vi "Shift.vi"() -> ()   [LabVIEW 2017]
uses:
  <vilib>/addons/database/Connection.llb/DB Tools Open Connec (String).vi
  <vilib>/addons/database/Auxilliary.llb/DB Tools Format Datetime String (Time Stamp).vi
  Global/Global 1.vi
  <vilib>/addons/database/NI_Database_API.lvlib
panel:
  out "error out":errorcluster
  in  "Cycle_time(s)":dbl
  out "x-y":dbl
  out "x-y 8":dbl
  out "x-y 7":dbl
  in  "INCLUDED 9":bool=TRUE
  in  "INCLUDED 8":bool=TRUE
  in  "INCLUDED 7":bool=TRUE
  in  "INCLUDED 6":bool=TRUE
  in  "INCLUDED 5":bool=TRUE
  in  "INCLUDED 4":bool=TRUE
  in  "INCLUDED 3":bool=TRUE
  in  "INCLUDED 2":bool=TRUE
  in  "INCLUDED":bool=TRUE
  in  "EXTRA SHIFT INCLUDED":bool=TRUE
  in  "Cancel Button":bool
  in  "Save Button":bool
  in  "Cluster 12":T1 {"1Start 4" format="%<%H:%M:%S>T"; "1Start 3" format="%<%H:%M:%S>T"; "1Start 2" format="%<%H:%M:%S>T"; "1Start" format="%<%H:%M:%S>T"}
  in  "Cluster 11":T1 {"1Start 4" format="%<%H:%M:%S>T"; "1Start 3" format="%<%H:%M:%S>T"; "1Start 2" format="%<%H:%M:%S>T"; "1Start" format="%<%H:%M:%S>T"}
  in  "Cluster 10":T1 {"1Start 4" format="%<%H:%M:%S>T"; "1Start 3" format="%<%H:%M:%S>T"; "1Start 2" format="%<%H:%M:%S>T"; "1Start" format="%<%H:%M:%S>T"}
  in  "Cluster 9":T1 {"1Start 4" format="%<%H:%M:%S>T"; "1Start 3" format="%<%H:%M:%S>T"; "1Start 2" format="%<%H:%M:%S>T"; "1Start" format="%<%H:%M:%S>T"}
  in  "Cluster 8":T2 {"1Start 8" format="%<%H:%M:%S>T"; "1Start 7" format="%<%H:%M:%S>T"; "1Start 6" format="%<%H:%M:%S>T"; "1Start 5" format="%<%H:%M:%S>T"; "1Start 4" format="%<%H:%M:%S>T"; "1Start 3" format="%<%H:%M:%S>T"; "1Start 2" format="%<%H:%M:%S>T"; "1Start" format="%<%H:%M:%S>T"}
  in  "Cluster 7":T2 {"1Start 8" format="%<%H:%M:%S>T"; "1Start 7" format="%<%H:%M:%S>T"; "1Start 6" format="%<%H:%M:%S>T"; "1Start 5" format="%<%H:%M:%S>T"; "1Start 4" format="%<%H:%M:%S>T"; "1Start 3" format="%<%H:%M:%S>T"; "1Start 2" format="%<%H:%M:%S>T"; "1Start" format="%<%H:%M:%S>T"}
  in  "Cluster 6":T2 {"1Start 8" format="%<%H:%M:%S>T"; "1Start 7" format="%<%H:%M:%S>T"; "1Start 6" format="%<%H:%M:%S>T"; "1Start 5" format="%<%H:%M:%S>T"; "1Start 4" format="%<%H:%M:%S>T"; "1Start 3" format="%<%H:%M:%S>T"; "1Start 2" format="%<%H:%M:%S>T"; "1Start" format="%<%H:%M:%S>T"}
  in  "Cluster 5":T2 {"1Start 8" format="%<%H:%M:%S>T"; "1Start 7" format="%<%H:%M:%S>T"; "1Start 6" format="%<%H:%M:%S>T"; "1Start 5" format="%<%H:%M:%S>T"; "1Start 4" format="%<%H:%M:%S>T"; "1Start 3" format="%<%H:%M:%S>T"; "1Start 2" format="%<%H:%M:%S>T"; "1Start" format="%<%H:%M:%S>T"}
  in  "Blank Button":bool
  in  "Cluster 4":T3 {"1Start 6" format="%<%H:%M:%S>T"; "1Start 5" format="%<%H:%M:%S>T"; "1Start 4" format="%<%H:%M:%S>T"; "1Start 3" format="%<%H:%M:%S>T"; "1Start 2" format="%<%H:%M:%S>T"; "1Start" format="%<%H:%M:%S>T"}
  in  "Cluster 3":T3 {"1Start 6" format="%<%H:%M:%S>T"; "1Start 5" format="%<%H:%M:%S>T"; "1Start 4" format="%<%H:%M:%S>T"; "1Start 3" format="%<%H:%M:%S>T"; "1Start 2" format="%<%H:%M:%S>T"; "1Start" format="%<%H:%M:%S>T"}
  in  "Cluster 2":T3 {"1Start 2" format="%<%H:%M:%S>T"; "1Start" format="%<%H:%M:%S>T"; "1Start 6" format="%<%H:%M:%S>T"; "1Start 5" format="%<%H:%M:%S>T"; "1Start 4" format="%<%H:%M:%S>T"; "1Start 3" format="%<%H:%M:%S>T"}
  in  "Cluster":T3 {"1Start 6" format="%<%H:%M:%S>T"; "1Start 5" format="%<%H:%M:%S>T"; "1Start 4" format="%<%H:%M:%S>T"; "1Start 3" format="%<%H:%M:%S>T"; "1Start 2" format="%<%H:%M:%S>T"; "1Start" format="%<%H:%M:%S>T"}
  # "SHIFT SETTING"
  # "EXTRA SHIFT"
  # "X"
  # "Y"
  # "A"
  # "B"
  # "C"
  # "D"
  # "BREAK 3"
  # "START"
  # "END"
  # "BREAK 2"
  # "START"
  # "END"
  # "BREAK 1"
  # "START"
  # "END"
  # "SHIFT IN DAY"
  # "CODE"
  # "START"
  # "END"
  # "A"
  # "B"
  # "C"
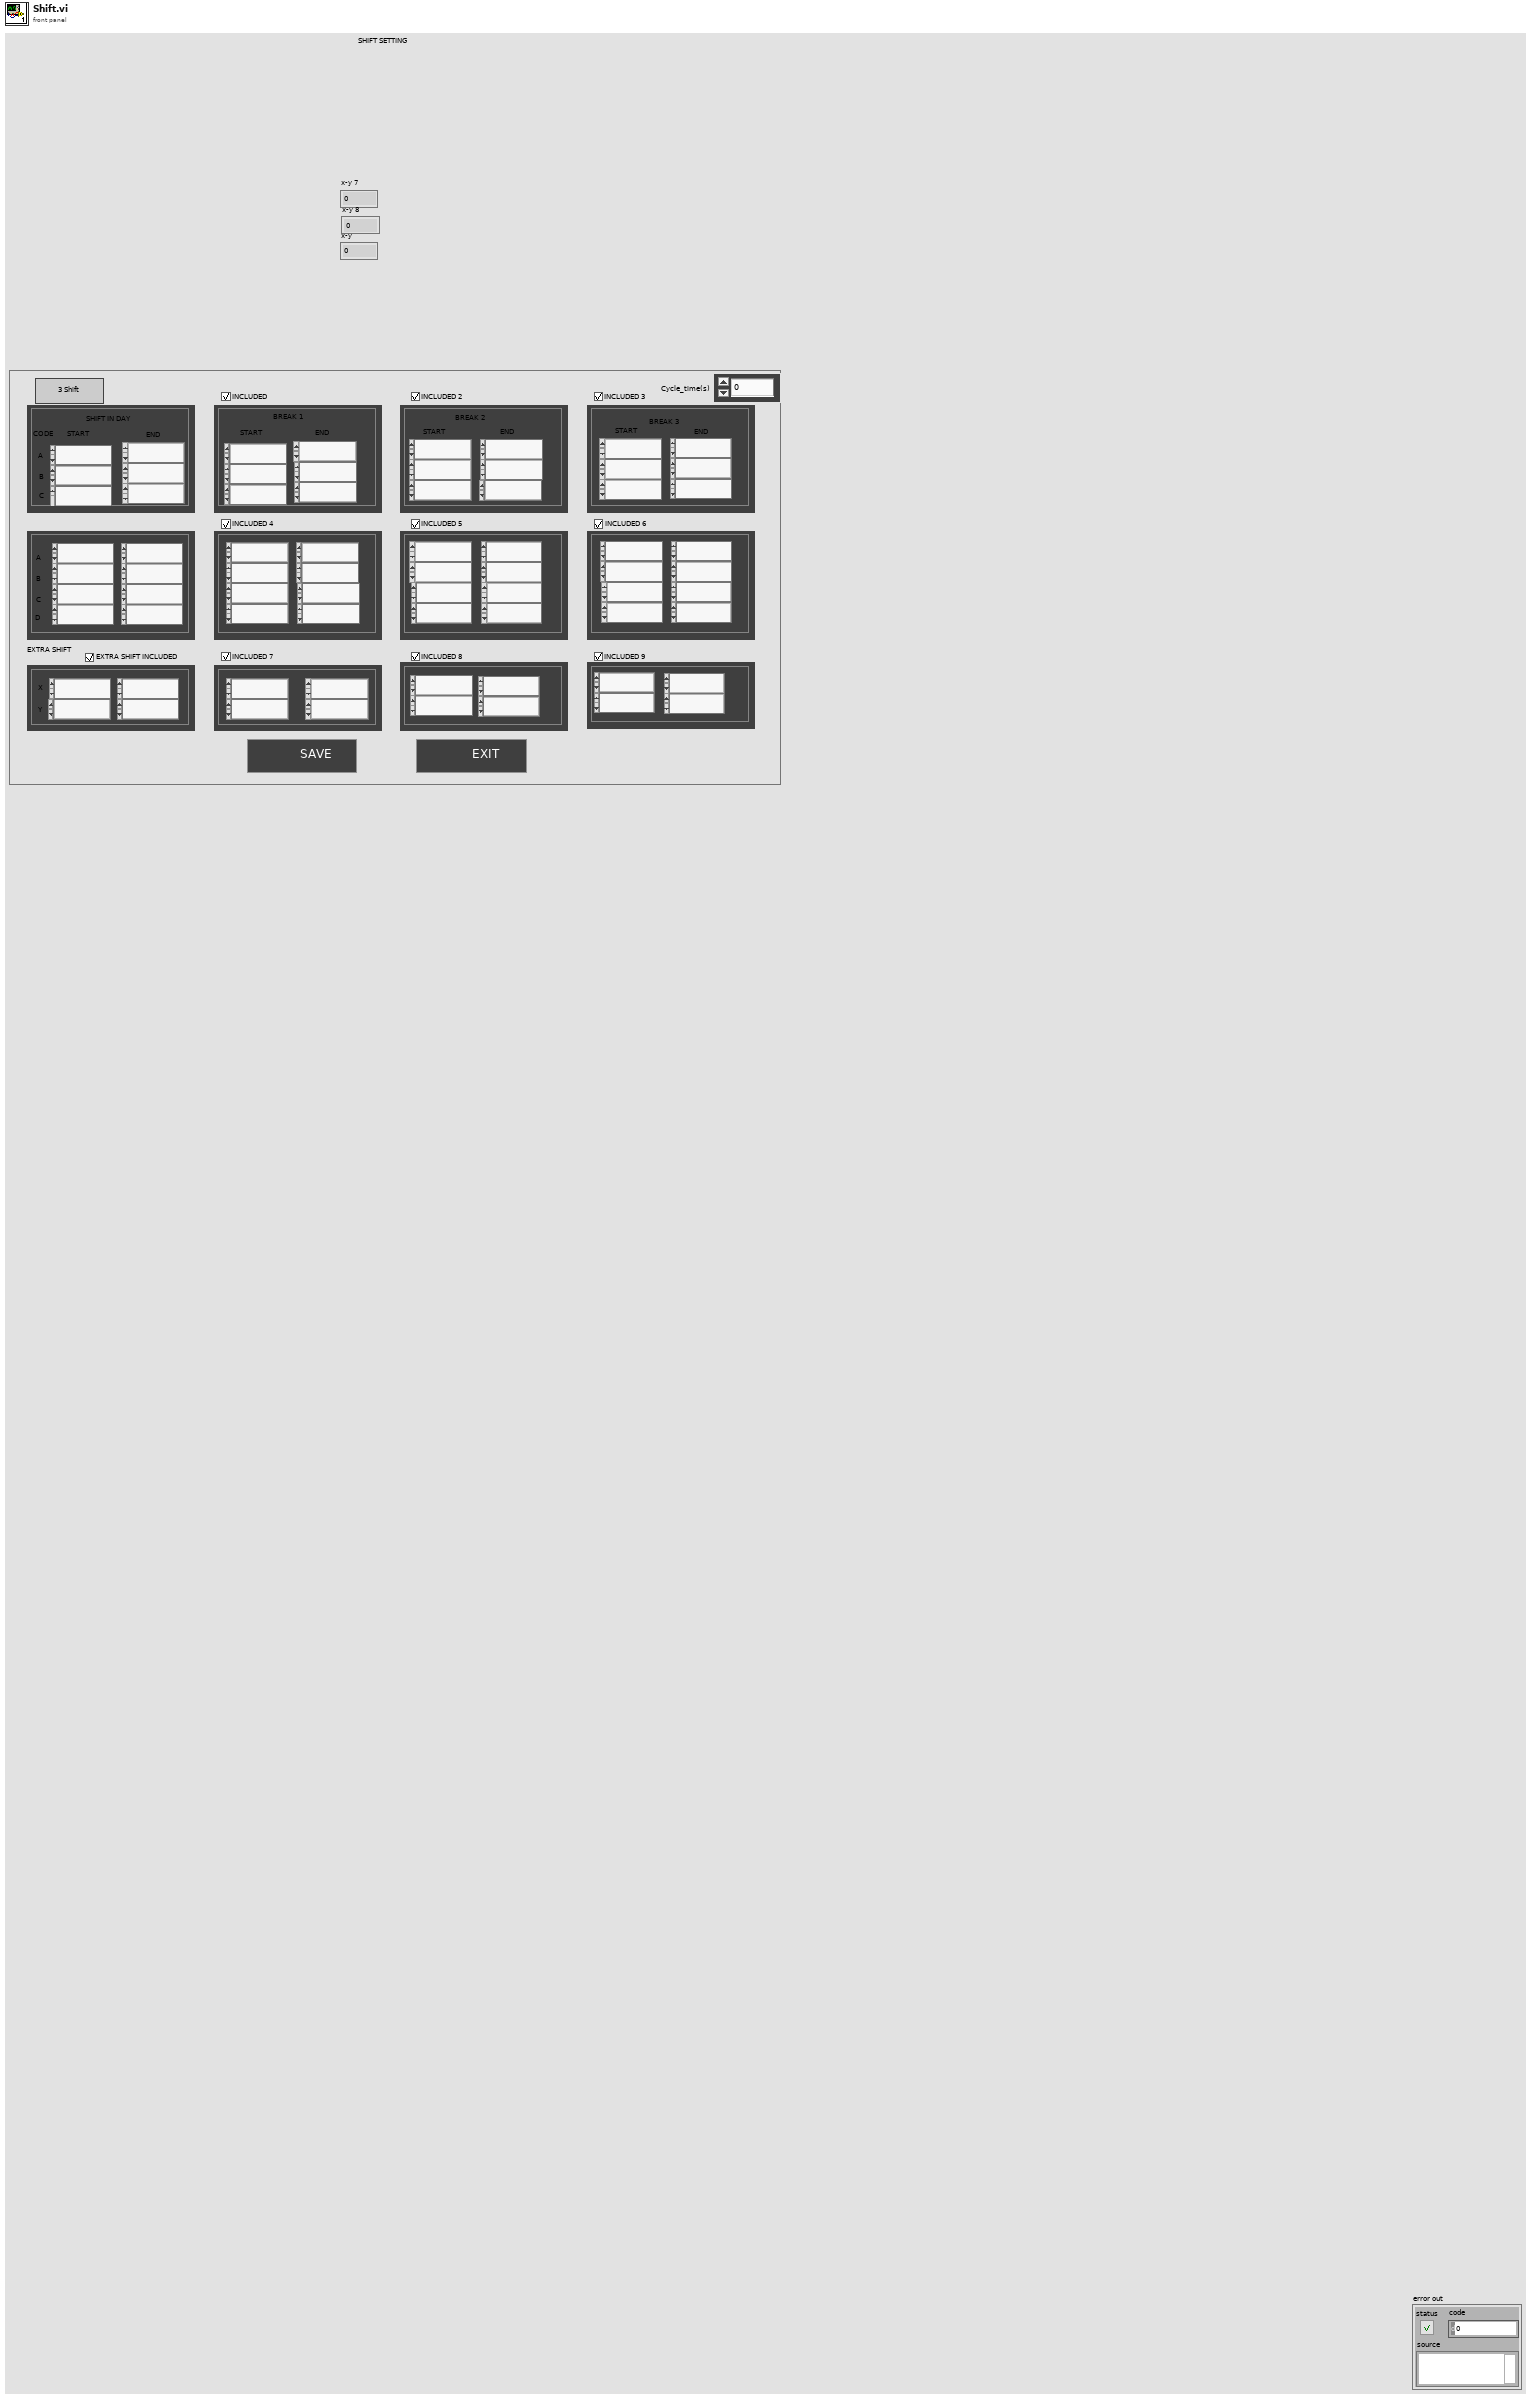
[diagram p1: front panel]
types:
  T1 = cluster{"1Start":timestamp, "1Start 2":timestamp, "1Start 3":timestamp, "1Start 4":timestamp}
  T2 = cluster{"1Start":timestamp, "1Start 2":timestamp, "1Start 3":timestamp, "1Start 4":timestamp, "1Start 5":timestamp, "1Start 6":timestamp, "1Start 7":timestamp, "1Start 8":timestamp}
  T3 = cluster{"1Start":timestamp, "1Start 2":timestamp, "1Start 3":timestamp, "1Start 4":timestamp, "1Start 5":timestamp, "1Start 6":timestamp}
  T4 = typedef "NI_Database_API.lvlib/Conn ObjectReference.ctl" = refnum<k1>
  T5 = cluster{"Time Stamp Out[0]":timestamp, "Time Stamp Out[1]":timestamp, "Time Stamp Out[2]":timestamp, "Time Stamp Out[3]":timestamp, "Time Stamp Out[4]":timestamp, "Time Stamp Out[5]":timestamp}
  T6 = cluster{"Time Stamp Out[0]":timestamp, "Time Stamp Out[1]":timestamp, "Time Stamp Out[2]":timestamp, "Time Stamp Out[3]":timestamp}
  T7 = cluster{"Time Stamp Out[0]":timestamp, "Time Stamp Out[1]":timestamp, "Time Stamp Out[2]":timestamp, "Time Stamp Out[3]":timestamp, "Time Stamp Out[4]":timestamp, "Time Stamp Out[5]":timestamp, "Time Stamp Out[6]":timestamp, "Time Stamp Out[7]":timestamp}
  T8 = cluster{"INCLUDED 9":bool, "date/time string":string, "date/time string":string, "date/time string":string, "date/time string":string}
  T9 = cluster{"INCLUDED 7":bool, "date/time string":string, "date/time string":string, "date/time string":string, "date/time string":string}
  T10 = cluster{"EXTRA SHIFT INCLUDED":bool, "date/time string":string, "date/time string":string, "date/time string":string, "date/time string":string}
  T11 = cluster{"INCLUDED 8":bool, "date/time string":string, "date/time string":string, "date/time string":string, "date/time string":string}
  T12 = cluster{"Blank Button":bool, "date/time string":string, "date/time string":string, "date/time string":string, "date/time string":string, "date/time string":string, "date/time string":string}
  T13 = cluster{"INCLUDED":bool, "date/time string":string, "date/time string":string, "date/time string":string, "date/time string":string, "date/time string":string, "date/time string":string}
  T14 = cluster{"INCLUDED 4":bool, "date/time string":string, "date/time string":string, "date/time string":string, "date/time string":string, "date/time string":string, "date/time string":string, "date/time string":string, "date/time string":string}
  T15 = cluster{"date/time string":string, "date/time string":string, "date/time string":string, "date/time string":string, "date/time string":string, "date/time string":string, "date/time string":string, "date/time string":string}
  T16 = cluster{"INCLUDED 6":bool, "date/time string":string, "date/time string":string, "date/time string":string, "date/time string":string, "date/time string":string, "date/time string":string, "date/time string":string, "date/time string":string}
  T17 = cluster{"INCLUDED 5":bool, "date/time string":string, "date/time string":string, "date/time string":string, "date/time string":string, "date/time string":string, "date/time string":string, "date/time string":string, "date/time string":string}
  T18 = cluster{"INCLUDED 2":bool, "date/time string":string, "date/time string":string, "date/time string":string, "date/time string":string, "date/time string":string, "date/time string":string}
  T19 = cluster{"INCLUDED 3":bool, "date/time string":string, "date/time string":string, "date/time string":string, "date/time string":string, "date/time string":string, "date/time string":string}
  T20 = enum32{"invalid app kind", "Development System", "Run Time System", "Student Edition", "Embedded LabVIEW", "Evaluation", "Custom"}
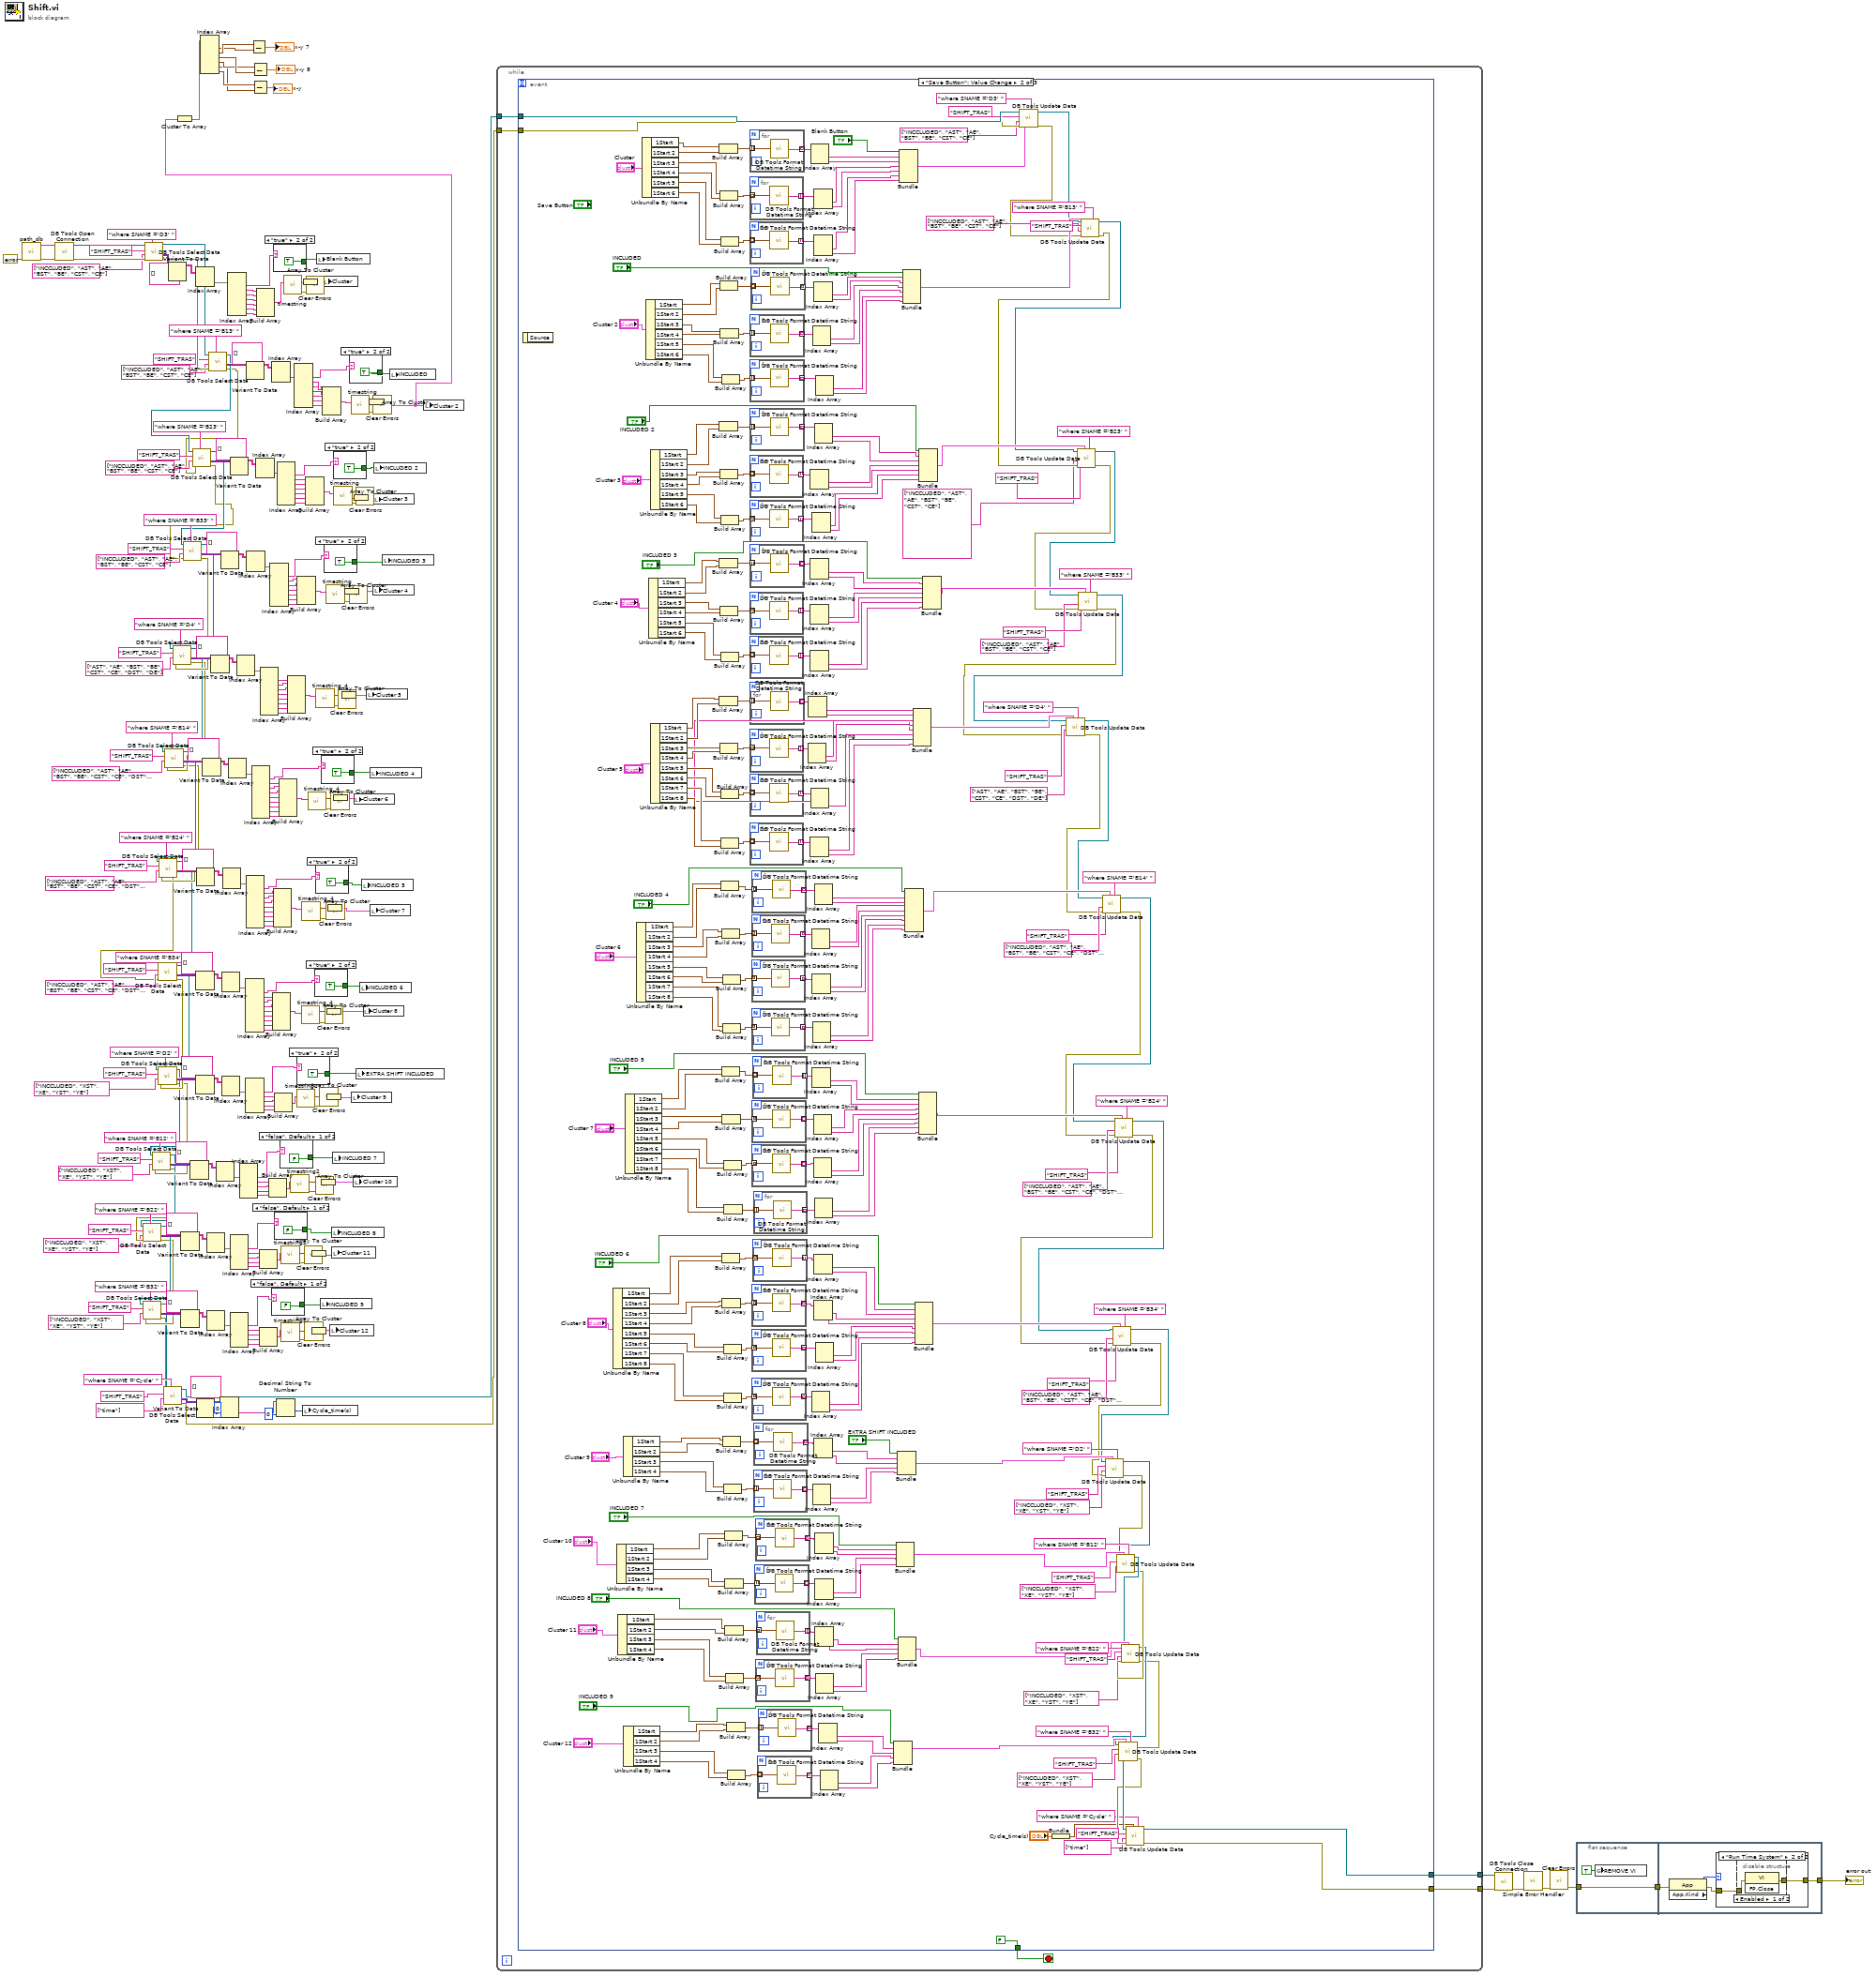
[diagram p0: block diagram]
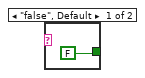
[diagram p4: hidden frame]
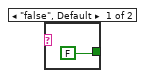
[diagram p5: hidden frame]
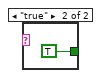
[diagram p6: hidden frame]
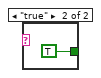
[diagram p7: hidden frame]
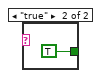
[diagram p8: hidden frame]
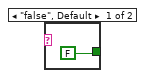
[diagram p9: hidden frame]
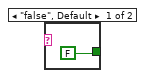
[diagram p10: hidden frame]
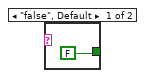
[diagram p11: hidden frame]
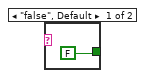
[diagram p12: hidden frame]
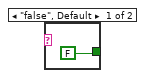
[diagram p13: hidden frame]
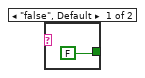
[diagram p14: hidden frame]
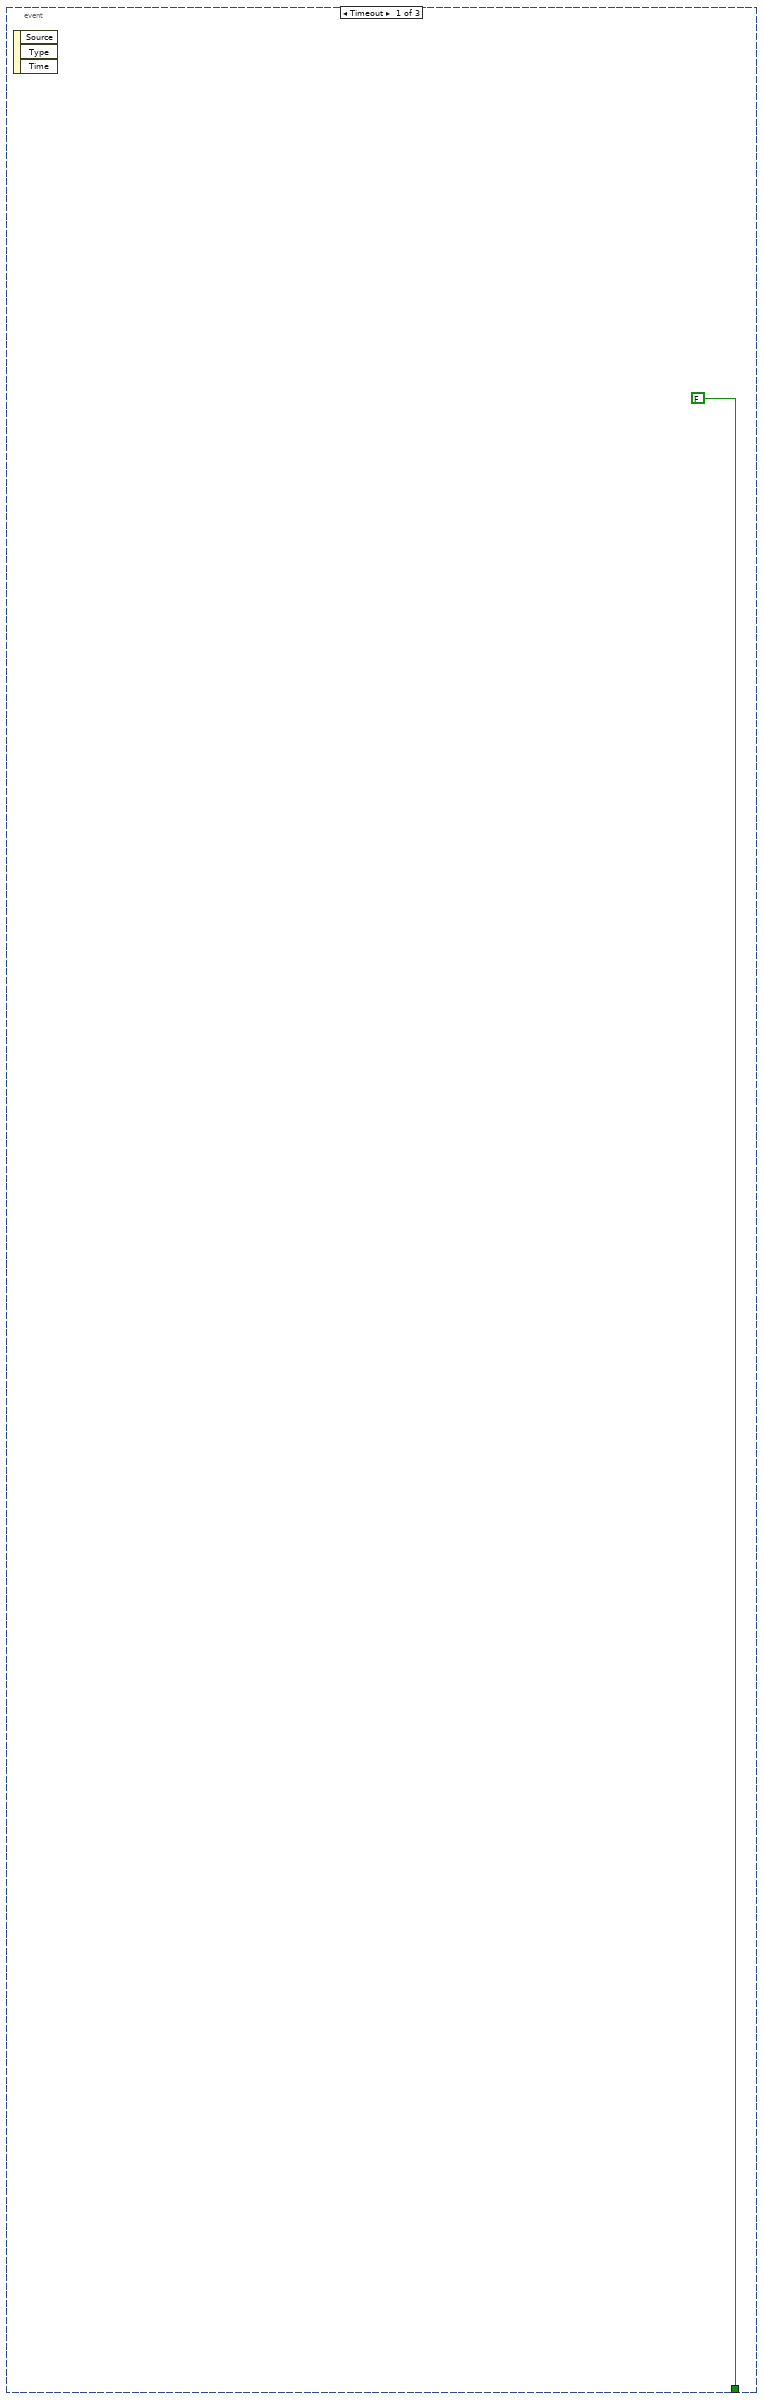
[diagram p15: hidden frame]
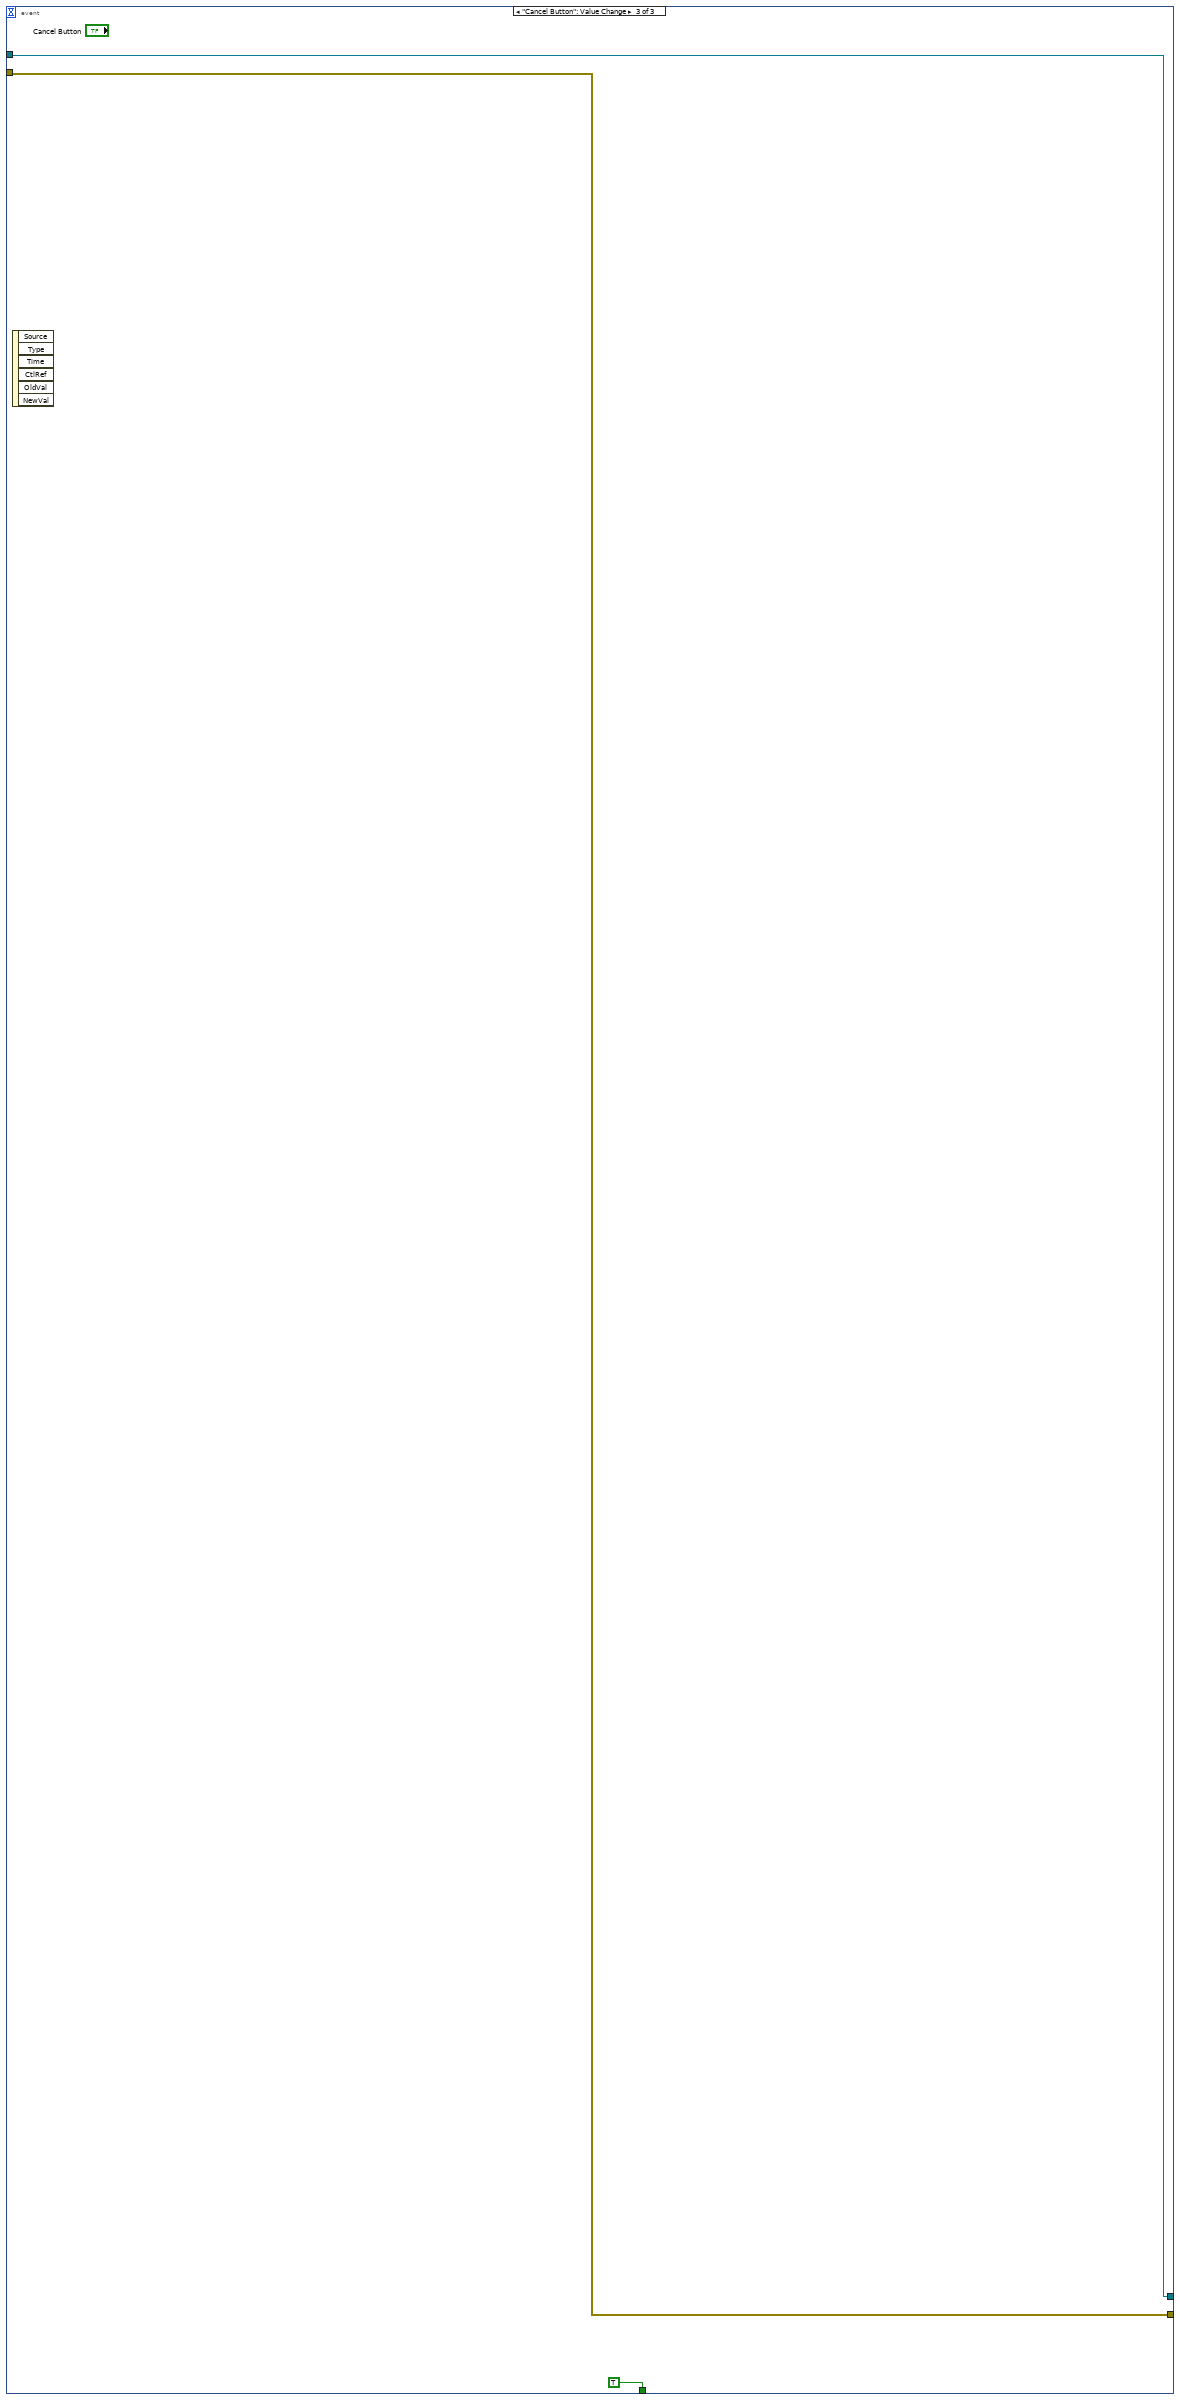
[diagram p16: hidden frame]
diagram:
  n1 = call "path_db.vi"("error in"=errorcluster {"status"=FALSE, "code"=0, "source"=""}) -> ("error out"=w284:errorcluster, "resulting string"=w285:string)  [unwired: 9 in]
  n2 = call-poly <vilib>:"DB Tools Open Connection.vi"("error in (no error)"=w284, "connection information"=w285) -> ("error out"=w281:errorcluster, "connection reference"=w280:T4)  [unwired: 6 in]
  n3 = call <vilib>:"DB Tools Select Data.vi"("condition"="where SNAME ='D3' ", "error in (no error)"=w281, "columns"=string[] ["INCCLUDED", "AST", "AE", "BST", "BE", "CST", "CE"], "table"="SHIFT_TRAS", "connection reference"=w280) -> ("error out"=w272:errorcluster, "data"=w277:variant[][], "connection reference out"=w271:T4)  [unwired: 1 in]
  n4 = Variant To Data(type=string[][] [], Variant=w277) -> (data=w275:string[][])  [unwired: 1 in, 1 out]
  n5 = Index Array(array=w275) -> (element=w43:string[])  [unwired: 2 in]
  n6 = call <vilib>:"DB Tools Select Data.vi"("condition"="where SNAME ='B13' ", "error in (no error)"=w272, "columns"=string[] ["INCCLUDED", "AST", "AE", "BST", "BE", "CST", "CE"], "table"="SHIFT_TRAS", "connection reference"=w271) -> ("error out"=w62:errorcluster, "data"=w267:variant[][], "connection reference out"=w217:T4)  [unwired: 1 in]
  n7 = call <vilib>:"DB Tools Select Data.vi"("condition"="where SNAME ='B23' ", "error in (no error)"=w62, "columns"=string[] ["INCCLUDED", "AST", "AE", "BST", "BE", "CST", "CE"], "table"="SHIFT_TRAS", "connection reference"=w217) -> ("error out"=w215:errorcluster, "data"=w241:variant[][], "connection reference out"=w216:T4)  [unwired: 1 in]
  n8 = call <vilib>:"DB Tools Select Data.vi"("condition"="where SNAME ='B33' ", "error in (no error)"=w215, "columns"=string[] ["INCCLUDED", "AST", "AE", "BST", "BE", "CST", "CE"], "table"="SHIFT_TRAS", "connection reference"=w216) -> ("error out"=w195:errorcluster, "data"=w234:variant[][], "connection reference out"=w196:T4)  [unwired: 1 in]
  n9 = call <vilib>:"DB Tools Select Data.vi"("condition"="where SNAME ='D4' ", "error in (no error)"=w195, "columns"=string[] ["AST", "AE", "BST", "BE", "CST", "CE", "DST", "DE"], "table"="SHIFT_TRAS", "connection reference"=w196) -> ("error out"=w75:errorcluster, "data"=w203:variant[][], "connection reference out"=w76:T4)  [unwired: 1 in]
  n10 = call <vilib>:"DB Tools Select Data.vi"("condition"="where SNAME ='B14' ", "error in (no error)"=w75, "columns"=string[] ["INCCLUDED", "AST", "AE", "BST", "BE", "CST", "CE", "DST", "DE"], "table"="SHIFT_TRAS", "connection reference"=w76) -> ("error out"=w73:errorcluster, "data"=w190:variant[][], "connection reference out"=w74:T4)  [unwired: 1 in]
  n11 = call <vilib>:"DB Tools Select Data.vi"("condition"="where SNAME ='B24' ", "error in (no error)"=w73, "columns"=string[] ["INCCLUDED", "AST", "AE", "BST", "BE", "CST", "CE", "DST", "DE"], "table"="SHIFT_TRAS", "connection reference"=w74) -> ("error out"=w71:errorcluster, "data"=w161:variant[][], "connection reference out"=w72:T4)  [unwired: 1 in]
  n12 = call <vilib>:"DB Tools Select Data.vi"("condition"="where SNAME ='B34' ", "error in (no error)"=w71, "columns"=string[] ["INCCLUDED", "AST", "AE", "BST", "BE", "CST", "CE", "DST", "DE"], "table"="SHIFT_TRAS", "connection reference"=w72) -> ("error out"=w69:errorcluster, "data"=w152:variant[][], "connection reference out"=w70:T4)  [unwired: 1 in]
  n13 = call <vilib>:"DB Tools Select Data.vi"("condition"="where SNAME ='D2' ", "error in (no error)"=w69, "columns"=string[] ["INCCLUDED", "XST", "XE", "YST", "YE"], "table"="SHIFT_TRAS", "connection reference"=w70) -> ("error out"=w67:errorcluster, "data"=w129:variant[][], "connection reference out"=w68:T4)  [unwired: 1 in]
  n14 = call <vilib>:"DB Tools Select Data.vi"("condition"="where SNAME ='B12' ", "error in (no error)"=w67, "columns"=string[] ["INCCLUDED", "XST", "XE", "YST", "YE"], "table"="SHIFT_TRAS", "connection reference"=w68) -> ("error out"=w65:errorcluster, "data"=w115:variant[][], "connection reference out"=w66:T4)  [unwired: 1 in]
  n15 = call <vilib>:"DB Tools Select Data.vi"("condition"="where SNAME ='B22' ", "error in (no error)"=w65, "columns"=string[] ["INCCLUDED", "XST", "XE", "YST", "YE"], "table"="SHIFT_TRAS", "connection reference"=w66) -> ("error out"=w63:errorcluster, "data"=w104:variant[][], "connection reference out"=w64:T4)  [unwired: 1 in]
  n16 = call <vilib>:"DB Tools Select Data.vi"("condition"="where SNAME ='B32' ", "error in (no error)"=w63, "columns"=string[] ["INCCLUDED", "XST", "XE", "YST", "YE"], "table"="SHIFT_TRAS", "connection reference"=w64) -> ("error out"=w14:errorcluster, "data"=w91:variant[][], "connection reference out"=w15:T4)  [unwired: 1 in]
  n17 = call <vilib>:"DB Tools Select Data.vi"("condition"="where SNAME ='Cycle' ", "error in (no error)"=w14, "columns"=string[] ["time"], "table"="SHIFT_TRAS", "connection reference"=w15) -> ("error out"=w13:errorcluster, "data"=w19:variant[][], "connection reference out"=w12:T4)  [unwired: 1 in]
  n18 = Variant To Data(type=string[][] [], Variant=w104) -> (data=w106:string[][])  [unwired: 1 in, 1 out]
  n19 = Variant To Data(type=string[][] [], Variant=w91) -> (data=w89:string[][])  [unwired: 1 in, 1 out]
  n20 = Variant To Data(type=string[][] [], Variant=w115) -> (data=w113:string[][])  [unwired: 1 in, 1 out]
  n21 = Variant To Data(type=string[][] [], Variant=w152) -> (data=w150:string[][])  [unwired: 1 in, 1 out]
  n22 = Variant To Data(type=string[][] [], Variant=w129) -> (data=w131:string[][])  [unwired: 1 in, 1 out]
  n23 = Variant To Data(type=string[][] [], Variant=w161) -> (data=w163:string[][])  [unwired: 1 in, 1 out]
  n24 = Variant To Data(type=string[][] [], Variant=w19) -> (data=w17:string[][])  [unwired: 1 in, 1 out]
  n25 = Variant To Data(type=string[][] [], Variant=w190) -> (data=w188:string[][])  [unwired: 1 in, 1 out]
  n26 = Index Array(array=w106) -> (element=w107:string[])  [unwired: 2 in]
  n27 = Index Array(array=w89) -> (element=w88:string[])  [unwired: 2 in]
  n28 = Variant To Data(type=string[][] [], Variant=w203) -> (data=w205:string[][])  [unwired: 1 in, 1 out]
  n29 = Index Array(array=w113) -> (element=w112:string[])  [unwired: 2 in]
  n30 = Index Array(array=w17, index (row)=0, index (col)=0 ("disabled index (col)")) -> (element=w9:string)
  n31 = Variant To Data(type=string[][] [], Variant=w234) -> (data=w232:string[][])  [unwired: 1 in, 1 out]
  n32 = Index Array(array=w150) -> (element=w149:string[])  [unwired: 2 in]
  n33 = Index Array(array=w131) -> (element=w132:string[])  [unwired: 2 in]
  n34 = Index Array(array=w163) -> (element=w164:string[])  [unwired: 2 in]
  n35 = Index Array(array=w43) -> (element #1=w35:string, element #2=w41:string, element #3=w40:string, element #4=w39:string, element #5=w38:string, element #6=w37:string, element #7=w36:string)  [unwired: 7 in]
  n36 = Index Array(array=w188) -> (element=w187:string[])  [unwired: 2 in]
  n37 = Variant To Data(type=string[][] [], Variant=w241) -> (data=w243:string[][])  [unwired: 1 in, 1 out]
  n38 = Index Array(array=w107) -> (element #1=w84:string, element #2=w100:string, element #3=w101:string, element #4=w99:string, element #5=w98:string)  [unwired: 5 in]
  n39 = Index Array(array=w88) -> (element #1=w83:string, element #2=w95:string, element #3=w94:string, element #4=w96:string, element #5=w97:string)  [unwired: 5 in]
  n40 = Index Array(array=w205) -> (element=w206:string[])  [unwired: 2 in]
  n41 = Index Array(array=w112) -> (element #1=w85:string, element #2=w119:string, element #3=w118:string, element #4=w120:string, element #5=w121:string)  [unwired: 5 in]
  n42 = Index Array(array=w149) -> (element #1=w139:string, element #2=w156:string, element #3=w148:string, element #4=w147:string, element #5=w146:string, element #6=w145:string, element #7=w144:string, element #8=w143:string, element #9=w155:string)  [unwired: 9 in]
  n43 = Index Array(array=w132) -> (element #1=w45:string, element #2=w125:string, element #3=w126:string, element #4=w123:string, element #5=w122:string)  [unwired: 5 in]
  n44 = Variant To Data(type=string[][] [], Variant=w267) -> (data=w265:string[][])  [unwired: 1 in, 1 out]
  n45 = Index Array(array=w164) -> (element #1=w174:string, element #2=w157:string, element #3=w165:string, element #4=w166:string, element #5=w167:string, element #6=w168:string, element #7=w169:string, element #8=w170:string, element #9=w158:string)  [unwired: 9 in]
  n46 = Index Array(array=w232) -> (element=w231:string[])  [unwired: 2 in]
  n47 = Index Array(array=w187) -> (element #1=w176:string, element #2=w194:string, element #3=w186:string, element #4=w185:string, element #5=w184:string, element #6=w183:string, element #7=w182:string, element #8=w181:string, element #9=w193:string)  [unwired: 9 in]
  n48 = Index Array(array=w243) -> (element=w244:string[])  [unwired: 2 in]
  n49 = Build Array(w41, w40, w39, w38, w37, w36) -> (w42:string[])
  n50 = Build Array(w100, w101, w99, w98) -> (w108:string[])
  n51 = Build Array(w95, w94, w96, w97) -> (w87:string[])
  n52 = Index Array(array=w206) -> (element #1=w198:string, element #2=w207:string, element #3=w208:string, element #4=w209:string, element #5=w210:string, element #6=w211:string, element #7=w212:string, element #8=w199:string)  [unwired: 8 in]
  n53 = Build Array(w119, w118, w120, w121) -> (w111:string[])
  n54 = Index Array(array=w231) -> (element #1=w222:string, element #2=w230:string, element #3=w229:string, element #4=w228:string, element #5=w227:string, element #6=w226:string, element #7=w225:string)  [unwired: 7 in]
  n55 = Index Array(array=w265) -> (element=w264:string[])  [unwired: 2 in]
  n56 = case shown="\"false\", Default" w83 {
    tunnel: [FALSE TRUE] -> w78
    frame "false", Default {
    }
    frame "true" {
    }
  }
  n57 = Build Array(w156, w148, w147, w146, w145, w144, w143, w155) -> (w142:string[])
  n58 = case shown="\"true\"" w35 {
    tunnel: [FALSE TRUE] -> w34
    frame "false", Default {
    }
    frame "true" {
    }
  }
  n59 = Build Array(w157, w165, w166, w167, w168, w169, w170, w158) -> (w171:string[])
  n60 = Build Array(w125, w126, w123, w122) -> (w133:string[])
  n61 = case shown="\"false\", Default" w84 {
    tunnel: [FALSE TRUE] -> w80
    frame "false", Default {
    }
    frame "true" {
    }
  }
  n62 = Decimal String To Number(string=w9, offset=0) -> (number=w8:i32)  [unwired: 1 in, 1 out]
  n63 = Index Array(array=w244) -> (element #1=w253:string, element #2=w245:string, element #3=w246:string, element #4=w247:string, element #5=w248:string, element #6=w249:string, element #7=w250:string)  [unwired: 7 in]
  n64 = Build Array(w194, w186, w185, w184, w183, w182, w181, w193) -> (w180:string[])
  n65 = case shown="\"false\", Default" w85 {
    tunnel: [FALSE TRUE] -> w81
    frame "false", Default {
    }
    frame "true" {
    }
  }
  n66 = call "timestring2.vi"("String Array In"=w108) -> ("error out"=w57:errorcluster, "Time Stamp Out"=w109:timestamp[])  [unwired: 9 in]
  n67 = call "timestring2.vi"("String Array In"=w87) -> ("error out"=w58:errorcluster, "Time Stamp Out"=w86:timestamp[])  [unwired: 9 in]
  n68 = call "timestring.vi"("String Array In"=w42) -> ("error out"=w47:errorcluster, "Time Stamp Out"=w274:timestamp[])  [unwired: 9 in]
  n69 = Build Array(w198, w207, w208, w209, w210, w211, w212, w199) -> (w213:string[])
  n70 = call "timestring2.vi"("String Array In"=w111) -> ("error out"=w56:errorcluster, "Time Stamp Out"=w110:timestamp[])  [unwired: 9 in]
  n71 = Index Array(array=w264) -> (element #1=w255:string, element #2=w263:string, element #3=w262:string, element #4=w261:string, element #5=w260:string, element #6=w259:string, element #7=w258:string)  [unwired: 7 in]
  n72 = call "timestring2.vi"("String Array In"=w133) -> ("error out"=w55:errorcluster, "Time Stamp Out"=w134:timestamp[])  [unwired: 9 in]
  n73 = Build Array(w230, w229, w228, w227, w226, w225) -> (w224:string[])
  n74 = case shown="\"true\"" w45 {
    tunnel: [FALSE TRUE] -> w44
    frame "false", Default {
    }
    frame "true" {
    }
  }
  n75 = Array To Cluster(array=w274) -> (cluster=w273:T5)
  n76 = call "timestring_4.vi"("String Array In"=w142) -> ("error out"=w54:errorcluster, "Time Stamp Out"=w141:timestamp[])  [unwired: 9 in]
  n77 = call "timestring_4.vi"("String Array In"=w171) -> ("error out"=w53:errorcluster, "Time Stamp Out"=w172:timestamp[])  [unwired: 9 in]
  n78 = local write "Cycle_time(s)"(w8) -> ()
  n79 = call <vilib>:"Clear Errors.vi"("error in (no error)"=w57) -> ()  [unwired: 5 in, 2 out]
  n80 = call <vilib>:"Clear Errors.vi"("error in (no error)"=w58) -> ()  [unwired: 5 in, 2 out]
  n81 = Build Array(w245, w246, w247, w248, w249, w250) -> (w251:string[])
  n82 = call <vilib>:"Clear Errors.vi"("error in (no error)"=w47) -> ()  [unwired: 5 in, 2 out]
  n83 = call "timestring_4.vi"("String Array In"=w180) -> ("error out"=w52:errorcluster, "Time Stamp Out"=w179:timestamp[])  [unwired: 9 in]
  n84 = Array To Cluster(array=w109) -> (cluster=w79:T6)
  n85 = Array To Cluster(array=w86) -> (cluster=w77:T6)
  n86 = case shown="\"true\"" w139 {
    tunnel: [FALSE TRUE] -> w135
    frame "false", Default {
    }
    frame "true" {
    }
  }
  n87 = case shown="\"true\"" w174 {
    tunnel: [FALSE TRUE] -> w136
    frame "false", Default {
    }
    frame "true" {
    }
  }
  n88 = call <vilib>:"Clear Errors.vi"("error in (no error)"=w56) -> ()  [unwired: 5 in, 2 out]
  n89 = call "timestring_4.vi"("String Array In"=w213) -> ("error out"=w51:errorcluster, "Time Stamp Out"=w214:timestamp[])  [unwired: 9 in]
  n90 = local write "Blank Button"(w34) -> ()
  n91 = Array To Cluster(array=w110) -> (cluster=w82:T6)
  n92 = call <vilib>:"Clear Errors.vi"("error in (no error)"=w55) -> ()  [unwired: 5 in, 2 out]
  n93 = local write "INCLUDED 9"(w78) -> ()
  n94 = case shown="\"true\"" w176 {
    tunnel: [FALSE TRUE] -> w175
    frame "false", Default {
    }
    frame "true" {
    }
  }
  n95 = local write "Cluster"(w273) -> ()
  n96 = Build Array(w263, w262, w261, w260, w259, w258) -> (w257:string[])
  n97 = case shown="\"true\"" w222 {
    tunnel: [FALSE TRUE] -> w219
    frame "false", Default {
    }
    frame "true" {
    }
  }
  n98 = Array To Cluster(array=w141) -> (cluster=w137:T7)
  n99 = call <vilib>:"Clear Errors.vi"("error in (no error)"=w54) -> ()  [unwired: 5 in, 2 out]
  n100 = Array To Cluster(array=w134) -> (cluster=w124:T6)
  n101 = Array To Cluster(array=w172) -> (cluster=w138:T7)
  n102 = call "timestring.vi"("String Array In"=w224) -> ("error out"=w50:errorcluster, "Time Stamp Out"=w223:timestamp[])  [unwired: 9 in]
  n103 = call <vilib>:"Clear Errors.vi"("error in (no error)"=w53) -> ()  [unwired: 5 in, 2 out]
  n104 = local write "Cluster 12"(w77) -> ()
  n105 = call <vilib>:"Clear Errors.vi"("error in (no error)"=w52) -> ()  [unwired: 5 in, 2 out]
  n106 = Array To Cluster(array=w179) -> (cluster=w178:T7)
  n107 = local write "INCLUDED 8"(w80) -> ()
  n108 = local write "Cluster 11"(w79) -> ()
  n109 = local write "INCLUDED 7"(w81) -> ()
  n110 = case shown="\"true\"" w253 {
    tunnel: [FALSE TRUE] -> w221
    frame "false", Default {
    }
    frame "true" {
    }
  }
  n111 = call "timestring.vi"("String Array In"=w251) -> ("error out"=w49:errorcluster, "Time Stamp Out"=w252:timestamp[])  [unwired: 9 in]
  n112 = call <vilib>:"Clear Errors.vi"("error in (no error)"=w51) -> ()  [unwired: 5 in, 2 out]
  n113 = Array To Cluster(array=w214) -> (cluster=w197:T7)
  n114 = Array To Cluster(array=w223) -> (cluster=w218:T5)
  n115 = call <vilib>:"Clear Errors.vi"("error in (no error)"=w50) -> ()  [unwired: 5 in, 2 out]
  n116 = case shown="\"true\"" w255 {
    tunnel: [FALSE TRUE] -> w254
    frame "false", Default {
    }
    frame "true" {
    }
  }
  n117 = call "timestring.vi"("String Array In"=w257) -> ("error out"=w48:errorcluster, "Time Stamp Out"=w256:timestamp[])  [unwired: 9 in]
  n118 = Array To Cluster(array=w252) -> (cluster=w220:T5)
  n119 = local write "Cluster 9"(w124) -> ()
  n120 = local write "Cluster 10"(w82) -> ()
  n121 = local write "Cluster 6"(w178) -> ()
  n122 = call <vilib>:"Clear Errors.vi"("error in (no error)"=w49) -> ()  [unwired: 5 in, 2 out]
  n123 = local write "EXTRA SHIFT INCLUDED"(w44) -> ()
  n124 = local write "INCLUDED 6"(w135) -> ()
  n125 = local write "INCLUDED 5"(w136) -> ()
  n126 = local write "Cluster 8"(w137) -> ()
  n127 = local write "Cluster 5"(w197) -> ()
  n128 = Array To Cluster(array=w256) -> (cluster=w32:T5)
  n129 = Cluster To Array(cluster=w32) -> (array=w31:timestamp[])
  n130 = Index Array(array=w31) -> (element #1=w29:timestamp, element #2=w30:timestamp, element #3=w27:timestamp, element #4=w26:timestamp, element #5=w23:timestamp, element #6=w24:timestamp)  [unwired: 6 in]
  n131 = Subtract(x=w30, y=w29) -> (x-y=→"x-y 7":dbl)
  n132 = Subtract(x=w26, y=w27) -> (x-y=→"x-y 8":dbl)
  n133 = Subtract(x=w24, y=w23) -> (x-y=→"x-y":dbl)
  n134 = local write "INCLUDED 4"(w175) -> ()
  n135 = local write "Cluster 7"(w138) -> ()
  n136 = call <vilib>:"Clear Errors.vi"("error in (no error)"=w48) -> ()  [unwired: 5 in, 2 out]
  n137 = local write "Cluster 3"(w220) -> ()
  n138 = local write "Cluster 4"(w218) -> ()
  n139 = local write "INCLUDED 2"(w221) -> ()
  n140 = local write "INCLUDED 3"(w219) -> ()
  n141 = local write "INCLUDED"(w254) -> ()
  n142 = local write "Cluster 2"(w32) -> ()
  n143 = while {
    tunnel: w12 -> [w311]
    tunnel: w13 -> [w310]
    tunnel: [w309] -> w283
    tunnel: [w308] -> w282
    stop <- w312 stop-if-true
    n144 = event shown="[1] \"Save Button\": Value Change" {
      selector: _ -> [_ _ _]
      dyn-events: _ -> [_ _ _]
      timeout: _ -> [_ _ _]
      tunnel: [FALSE FALSE TRUE] -> w312
      tunnel: w311 -> [_ w444 w708]
      tunnel: w310 -> [_ w443 w707]
      tunnel: [_ w320 w708] -> w309
      tunnel: [_ w319 w707] -> w308
      event Timeout {
        n145 = event-data() -> ()  [unwired: 1 in, 3 out]
      }
      event "Save Button": Value Change {
        n146 = event-data() -> ()  [unwired: 1 in, 1 out]
        n147 = Unbundle By Name("Cluster 8") -> ("1Start"=w550:timestamp, "1Start 2"=w549:timestamp, "1Start 3"=w548:timestamp, "1Start 4"=w547:timestamp, "1Start 5"=w546:timestamp, "1Start 6"=w545:timestamp, "1Start 7"=w544:timestamp, "1Start 8"=w543:timestamp)
        n148 = Unbundle By Name("Cluster 10") -> ("1Start"=w528:timestamp, "1Start 2"=w527:timestamp, "1Start 3"=w526:timestamp, "1Start 4"=w525:timestamp)
        n149 = Unbundle By Name("Cluster 11") -> ("1Start"=w524:timestamp, "1Start 2"=w523:timestamp, "1Start 3"=w522:timestamp, "1Start 4"=w521:timestamp)
        n150 = Unbundle By Name("Cluster 9") -> ("1Start"=w536:timestamp, "1Start 2"=w535:timestamp, "1Start 3"=w534:timestamp, "1Start 4"=w533:timestamp)
        n151 = Unbundle By Name("Cluster 12") -> ("1Start"=w518:timestamp, "1Start 2"=w517:timestamp, "1Start 3"=w516:timestamp, "1Start 4"=w515:timestamp)
        n152 = Unbundle By Name("Cluster 7") -> ("1Start"=w563:timestamp, "1Start 2"=w562:timestamp, "1Start 3"=w561:timestamp, "1Start 4"=w560:timestamp, "1Start 5"=w559:timestamp, "1Start 6"=w558:timestamp, "1Start 7"=w557:timestamp, "1Start 8"=w556:timestamp)
        n153 = Unbundle By Name("Cluster 6") -> ("1Start"=w576:timestamp, "1Start 2"=w575:timestamp, "1Start 3"=w574:timestamp, "1Start 4"=w573:timestamp, "1Start 5"=w572:timestamp, "1Start 6"=w571:timestamp, "1Start 7"=w570:timestamp, "1Start 8"=w569:timestamp)
        n154 = Unbundle By Name("Cluster") -> ("1Start"=w631:timestamp, "1Start 2"=w630:timestamp, "1Start 3"=w627:timestamp, "1Start 4"=w626:timestamp, "1Start 5"=w625:timestamp, "1Start 6"=w624:timestamp)
        n155 = Unbundle By Name("Cluster 2") -> ("1Start"=w620:timestamp, "1Start 2"=w619:timestamp, "1Start 3"=w618:timestamp, "1Start 4"=w617:timestamp, "1Start 5"=w616:timestamp, "1Start 6"=w615:timestamp)
        n156 = Unbundle By Name("Cluster 4") -> ("1Start"=w600:timestamp, "1Start 2"=w599:timestamp, "1Start 3"=w598:timestamp, "1Start 4"=w597:timestamp, "1Start 5"=w596:timestamp, "1Start 6"=w595:timestamp)
        n157 = Unbundle By Name("Cluster 3") -> ("1Start"=w610:timestamp, "1Start 2"=w609:timestamp, "1Start 3"=w608:timestamp, "1Start 4"=w607:timestamp, "1Start 5"=w606:timestamp, "1Start 6"=w605:timestamp)
        n158 = Unbundle By Name("Cluster 5") -> ("1Start"=w589:timestamp, "1Start 2"=w588:timestamp, "1Start 3"=w587:timestamp, "1Start 4"=w586:timestamp, "1Start 5"=w585:timestamp, "1Start 6"=w584:timestamp, "1Start 7"=w583:timestamp, "1Start 8"=w582:timestamp)
        n159 = Build Array(w631, w630) -> (w633:timestamp[])
        n160 = Build Array(w610, w609) -> (w613:timestamp[])
        n161 = Build Array(w600, w599) -> (w601:timestamp[])
        n162 = Build Array(w589, w588) -> (w593:timestamp[])
        n163 = Build Array(w627, w626) -> (w629:timestamp[])
        n164 = Build Array(w620, w619) -> (w621:timestamp[])
        n165 = Build Array(w608, w607) -> (w612:timestamp[])
        n166 = Build Array(w598, w597) -> (w602:timestamp[])
        n167 = Build Array(w587, w586) -> (w592:timestamp[])
        n168 = Build Array(w618, w617) -> (w622:timestamp[])
        n169 = Build Array(w625, w624) -> (w628:timestamp[])
        n170 = Build Array(w606, w605) -> (w611:timestamp[])
        n171 = Build Array(w596, w595) -> (w603:timestamp[])
        n172 = Build Array(w585, w584) -> (w591:timestamp[])
        n173 = Build Array(w583, w582) -> (w590:timestamp[])
        n174 = Build Array(w576, w575) -> (w577:timestamp[])
        n175 = Build Array(w616, w615) -> (w623:timestamp[])
        n176 = Build Array(w574, w573) -> (w578:timestamp[])
        n177 = Build Array(w563, w562) -> (w567:timestamp[])
        n178 = Build Array(w550, w549) -> (w551:timestamp[])
        n179 = Build Array(w561, w560) -> (w566:timestamp[])
        n180 = Build Array(w548, w547) -> (w552:timestamp[])
        n181 = Build Array(w572, w571) -> (w579:timestamp[])
        n182 = Build Array(w570, w569) -> (w580:timestamp[])
        n183 = Build Array(w536, w535) -> (w538:timestamp[])
        n184 = Build Array(w559, w558) -> (w565:timestamp[])
        n185 = Build Array(w546, w545) -> (w553:timestamp[])
        n186 = Build Array(w544, w543) -> (w554:timestamp[])
        n187 = Build Array(w534, w533) -> (w537:timestamp[])
        n188 = Build Array(w557, w556) -> (w564:timestamp[])
        n189 = Build Array(w528, w527) -> (w531:timestamp[])
        n190 = Build Array(w526, w525) -> (w532:timestamp[])
        n191 = Build Array(w524, w523) -> (w530:timestamp[])
        n192 = Build Array(w522, w521) -> (w529:timestamp[])
        n193 = Build Array(w518, w517) -> (w519:timestamp[])
        n194 = Build Array(w516, w515) -> (w520:timestamp[])
        n195 = for {
          tunnel: w629 -> [w704] mode=indexing
          tunnel: [w703] -> w513 mode=indexing
          n196 = call-poly <vilib>:"DB Tools Format Datetime String.vi"("time stamp"=w704) -> ("date/time string"=w703:string)
        }
        n197 = for {
          tunnel: w628 -> [w702] mode=indexing
          tunnel: [w701] -> w512 mode=indexing
          n198 = call-poly <vilib>:"DB Tools Format Datetime String.vi"("time stamp"=w702) -> ("date/time string"=w701:string)
        }
        n199 = for {
          tunnel: w612 -> [w691] mode=indexing
          tunnel: [w692] -> w508 mode=indexing
          n200 = call-poly <vilib>:"DB Tools Format Datetime String.vi"("time stamp"=w691) -> ("date/time string"=w692:string)
        }
        n201 = for {
          tunnel: w611 -> [w689] mode=indexing
          tunnel: [w690] -> w506 mode=indexing
          n202 = call-poly <vilib>:"DB Tools Format Datetime String.vi"("time stamp"=w689) -> ("date/time string"=w690:string)
        }
        n203 = for {
          tunnel: w602 -> [w685] mode=indexing
          tunnel: [w686] -> w504 mode=indexing
          n204 = call-poly <vilib>:"DB Tools Format Datetime String.vi"("time stamp"=w685) -> ("date/time string"=w686:string)
        }
        n205 = for {
          tunnel: w603 -> [w683] mode=indexing
          tunnel: [w684] -> w503 mode=indexing
          n206 = call-poly <vilib>:"DB Tools Format Datetime String.vi"("time stamp"=w683) -> ("date/time string"=w684:string)
        }
        n207 = for {
          tunnel: w592 -> [w679] mode=indexing
          tunnel: [w680] -> w501 mode=indexing
          n208 = call-poly <vilib>:"DB Tools Format Datetime String.vi"("time stamp"=w679) -> ("date/time string"=w680:string)
        }
        n209 = for {
          tunnel: w591 -> [w677] mode=indexing
          tunnel: [w678] -> w500 mode=indexing
          n210 = call-poly <vilib>:"DB Tools Format Datetime String.vi"("time stamp"=w677) -> ("date/time string"=w678:string)
        }
        n211 = for {
          tunnel: w590 -> [w675] mode=indexing
          tunnel: [w676] -> w499 mode=indexing
          n212 = call-poly <vilib>:"DB Tools Format Datetime String.vi"("time stamp"=w675) -> ("date/time string"=w676:string)
        }
        n213 = for {
          tunnel: w633 -> [w706] mode=indexing
          tunnel: [w705] -> w514 mode=indexing
          n214 = call-poly <vilib>:"DB Tools Format Datetime String.vi"("time stamp"=w706) -> ("date/time string"=w705:string)
        }
        n215 = for {
          tunnel: w622 -> [w697] mode=indexing
          tunnel: [w698] -> w510 mode=indexing
          n216 = call-poly <vilib>:"DB Tools Format Datetime String.vi"("time stamp"=w697) -> ("date/time string"=w698:string)
        }
        n217 = for {
          tunnel: w623 -> [w695] mode=indexing
          tunnel: [w696] -> w507 mode=indexing
          n218 = call-poly <vilib>:"DB Tools Format Datetime String.vi"("time stamp"=w695) -> ("date/time string"=w696:string)
        }
        n219 = for {
          tunnel: w613 -> [w693] mode=indexing
          tunnel: [w694] -> w509 mode=indexing
          n220 = call-poly <vilib>:"DB Tools Format Datetime String.vi"("time stamp"=w693) -> ("date/time string"=w694:string)
        }
        n221 = for {
          tunnel: w601 -> [w687] mode=indexing
          tunnel: [w688] -> w505 mode=indexing
          n222 = call-poly <vilib>:"DB Tools Format Datetime String.vi"("time stamp"=w687) -> ("date/time string"=w688:string)
        }
        n223 = for {
          tunnel: w593 -> [w681] mode=indexing
          tunnel: [w682] -> w502 mode=indexing
          n224 = call-poly <vilib>:"DB Tools Format Datetime String.vi"("time stamp"=w681) -> ("date/time string"=w682:string)
        }
        n225 = for {
          tunnel: w621 -> [w699] mode=indexing
          tunnel: [w700] -> w511 mode=indexing
          n226 = call-poly <vilib>:"DB Tools Format Datetime String.vi"("time stamp"=w699) -> ("date/time string"=w700:string)
        }
        n227 = for {
          tunnel: w578 -> [w671] mode=indexing
          tunnel: [w672] -> w497 mode=indexing
          n228 = call-poly <vilib>:"DB Tools Format Datetime String.vi"("time stamp"=w671) -> ("date/time string"=w672:string)
        }
        n229 = for {
          tunnel: w579 -> [w669] mode=indexing
          tunnel: [w670] -> w496 mode=indexing
          n230 = call-poly <vilib>:"DB Tools Format Datetime String.vi"("time stamp"=w669) -> ("date/time string"=w670:string)
        }
        n231 = for {
          tunnel: w580 -> [w667] mode=indexing
          tunnel: [w668] -> w495 mode=indexing
          n232 = call-poly <vilib>:"DB Tools Format Datetime String.vi"("time stamp"=w667) -> ("date/time string"=w668:string)
        }
        n233 = for {
          tunnel: w577 -> [w673] mode=indexing
          tunnel: [w674] -> w498 mode=indexing
          n234 = call-poly <vilib>:"DB Tools Format Datetime String.vi"("time stamp"=w673) -> ("date/time string"=w674:string)
        }
        n235 = for {
          tunnel: w566 -> [w663] mode=indexing
          tunnel: [w664] -> w493 mode=indexing
          n236 = call-poly <vilib>:"DB Tools Format Datetime String.vi"("time stamp"=w663) -> ("date/time string"=w664:string)
        }
        n237 = for {
          tunnel: w565 -> [w661] mode=indexing
          tunnel: [w662] -> w492 mode=indexing
          n238 = call-poly <vilib>:"DB Tools Format Datetime String.vi"("time stamp"=w661) -> ("date/time string"=w662:string)
        }
        n239 = for {
          tunnel: w552 -> [w655] mode=indexing
          tunnel: [w656] -> w489 mode=indexing
          n240 = call-poly <vilib>:"DB Tools Format Datetime String.vi"("time stamp"=w655) -> ("date/time string"=w656:string)
        }
        n241 = for {
          tunnel: w553 -> [w653] mode=indexing
          tunnel: [w654] -> w488 mode=indexing
          n242 = call-poly <vilib>:"DB Tools Format Datetime String.vi"("time stamp"=w653) -> ("date/time string"=w654:string)
        }
        n243 = for {
          tunnel: w554 -> [w651] mode=indexing
          tunnel: [w652] -> w487 mode=indexing
          n244 = call-poly <vilib>:"DB Tools Format Datetime String.vi"("time stamp"=w651) -> ("date/time string"=w652:string)
        }
        n245 = for {
          tunnel: w567 -> [w665] mode=indexing
          tunnel: [w666] -> w494 mode=indexing
          n246 = call-poly <vilib>:"DB Tools Format Datetime String.vi"("time stamp"=w665) -> ("date/time string"=w666:string)
        }
        n247 = for {
          tunnel: w551 -> [w657] mode=indexing
          tunnel: [w658] -> w490 mode=indexing
          n248 = call-poly <vilib>:"DB Tools Format Datetime String.vi"("time stamp"=w657) -> ("date/time string"=w658:string)
        }
        n249 = for {
          tunnel: w564 -> [w659] mode=indexing
          tunnel: [w660] -> w491 mode=indexing
          n250 = call-poly <vilib>:"DB Tools Format Datetime String.vi"("time stamp"=w659) -> ("date/time string"=w660:string)
        }
        n251 = for {
          tunnel: w537 -> [w647] mode=indexing
          tunnel: [w648] -> w485 mode=indexing
          n252 = call-poly <vilib>:"DB Tools Format Datetime String.vi"("time stamp"=w647) -> ("date/time string"=w648:string)
        }
        n253 = for {
          tunnel: w538 -> [w649] mode=indexing
          tunnel: [w650] -> w486 mode=indexing
          n254 = call-poly <vilib>:"DB Tools Format Datetime String.vi"("time stamp"=w649) -> ("date/time string"=w650:string)
        }
        n255 = for {
          tunnel: w532 -> [w643] mode=indexing
          tunnel: [w644] -> w483 mode=indexing
          n256 = call-poly <vilib>:"DB Tools Format Datetime String.vi"("time stamp"=w643) -> ("date/time string"=w644:string)
        }
        n257 = for {
          tunnel: w531 -> [w645] mode=indexing
          tunnel: [w646] -> w484 mode=indexing
          n258 = call-poly <vilib>:"DB Tools Format Datetime String.vi"("time stamp"=w645) -> ("date/time string"=w646:string)
        }
        n259 = for {
          tunnel: w529 -> [w639] mode=indexing
          tunnel: [w640] -> w481 mode=indexing
          n260 = call-poly <vilib>:"DB Tools Format Datetime String.vi"("time stamp"=w639) -> ("date/time string"=w640:string)
        }
        n261 = for {
          tunnel: w530 -> [w641] mode=indexing
          tunnel: [w642] -> w482 mode=indexing
          n262 = call-poly <vilib>:"DB Tools Format Datetime String.vi"("time stamp"=w641) -> ("date/time string"=w642:string)
        }
        n263 = for {
          tunnel: w520 -> [w635] mode=indexing
          tunnel: [w636] -> w479 mode=indexing
          n264 = call-poly <vilib>:"DB Tools Format Datetime String.vi"("time stamp"=w635) -> ("date/time string"=w636:string)
        }
        n265 = for {
          tunnel: w519 -> [w637] mode=indexing
          tunnel: [w638] -> w480 mode=indexing
          n266 = call-poly <vilib>:"DB Tools Format Datetime String.vi"("time stamp"=w637) -> ("date/time string"=w638:string)
        }
        n267 = Index Array(array=w501) -> (element #1=w450:string, element #2=w449:string)  [unwired: 2 in]
        n268 = Index Array(array=w502) -> (element #1=w452:string, element #2=w451:string)  [unwired: 2 in]
        n269 = Index Array(array=w508) -> (element #1=w462:string, element #2=w461:string)  [unwired: 2 in]
        n270 = Index Array(array=w505) -> (element #1=w458:string, element #2=w457:string)  [unwired: 2 in]
        n271 = Index Array(array=w504) -> (element #1=w456:string, element #2=w455:string)  [unwired: 2 in]
        n272 = Index Array(array=w503) -> (element #1=w454:string, element #2=w453:string)  [unwired: 2 in]
        n273 = Index Array(array=w499) -> (element #1=w446:string, element #2=w445:string)  [unwired: 2 in]
        n274 = Index Array(array=w514) -> (element #1=w478:string, element #2=w477:string)  [unwired: 2 in]
        n275 = Index Array(array=w500) -> (element #1=w448:string, element #2=w447:string)  [unwired: 2 in]
        n276 = Index Array(array=w497) -> (element #1=w413:string, element #2=w412:string)  [unwired: 2 in]
        n277 = Index Array(array=w487) -> (element #1=w390:string, element #2=w389:string)  [unwired: 2 in]
        n278 = Index Array(array=w506) -> (element #1=w460:string, element #2=w459:string)  [unwired: 2 in]
        n279 = Index Array(array=w496) -> (element #1=w411:string, element #2=w410:string)  [unwired: 2 in]
        n280 = Index Array(array=w494) -> (element #1=w406:string, element #2=w405:string)  [unwired: 2 in]
        n281 = Index Array(array=w510) -> (element #1=w468:string, element #2=w467:string)  [unwired: 2 in]
        n282 = Index Array(array=w495) -> (element #1=w409:string, element #2=w408:string)  [unwired: 2 in]
        n283 = Index Array(array=w485) -> (element #1=w384:string, element #2=w383:string)  [unwired: 2 in]
        n284 = Index Array(array=w493) -> (element #1=w404:string, element #2=w403:string)  [unwired: 2 in]
        n285 = Index Array(array=w492) -> (element #1=w402:string, element #2=w401:string)  [unwired: 2 in]
        n286 = Index Array(array=w513) -> (element #1=w476:string, element #2=w475:string)  [unwired: 2 in]
        n287 = Index Array(array=w512) -> (element #1=w474:string, element #2=w473:string)  [unwired: 2 in]
        n288 = Index Array(array=w511) -> (element #1=w470:string, element #2=w469:string)  [unwired: 2 in]
        n289 = Index Array(array=w490) -> (element #1=w396:string, element #2=w395:string)  [unwired: 2 in]
        n290 = Index Array(array=w489) -> (element #1=w394:string, element #2=w393:string)  [unwired: 2 in]
        n291 = Index Array(array=w486) -> (element #1=w386:string, element #2=w385:string)  [unwired: 2 in]
        n292 = Index Array(array=w509) -> (element #1=w464:string, element #2=w463:string)  [unwired: 2 in]
        n293 = Index Array(array=w498) -> (element #1=w415:string, element #2=w414:string)  [unwired: 2 in]
        n294 = Index Array(array=w491) -> (element #1=w400:string, element #2=w399:string)  [unwired: 2 in]
        n295 = Index Array(array=w484) -> (element #1=w382:string, element #2=w381:string)  [unwired: 2 in]
        n296 = Index Array(array=w483) -> (element #1=w380:string, element #2=w379:string)  [unwired: 2 in]
        n297 = Index Array(array=w482) -> (element #1=w378:string, element #2=w377:string)  [unwired: 2 in]
        n298 = Index Array(array=w507) -> (element #1=w466:string, element #2=w465:string)  [unwired: 2 in]
        n299 = Index Array(array=w488) -> (element #1=w392:string, element #2=w391:string)  [unwired: 2 in]
        n300 = Index Array(array=w481) -> (element #1=w376:string, element #2=w375:string)  [unwired: 2 in]
        n301 = Index Array(array=w480) -> (element #1=w374:string, element #2=w373:string)  [unwired: 2 in]
        n302 = Index Array(array=w479) -> (element #1=w372:string, element #2=w371:string)  [unwired: 2 in]
        n303 = Bundle("INCLUDED 9"="INCLUDED 9", "date/time string"=w374, "date/time string"=w373, "date/time string"=w372, "date/time string"=w371) -> (w360:T8)  [unwired: 1 in]
        n304 = Bundle("INCLUDED 7"="INCLUDED 7", "date/time string"=w382, "date/time string"=w381, "date/time string"=w380, "date/time string"=w379) -> (w366:T9)  [unwired: 1 in]
        n305 = Bundle("EXTRA SHIFT INCLUDED"="EXTRA SHIFT INCLUDED", "date/time string"=w386, "date/time string"=w385, "date/time string"=w384, "date/time string"=w383) -> (w370:T10)  [unwired: 1 in]
        n306 = Bundle("INCLUDED 8"="INCLUDED 8", "date/time string"=w378, "date/time string"=w377, "date/time string"=w376, "date/time string"=w375) -> (w363:T11)  [unwired: 1 in]
        n307 = Bundle("Blank Button"="Blank Button", "date/time string"=w478, "date/time string"=w477, "date/time string"=w476, "date/time string"=w475, "date/time string"=w474, "date/time string"=w473) -> (w472:T12)  [unwired: 1 in]
        n308 = Bundle("INCLUDED"="INCLUDED", "date/time string"=w470, "date/time string"=w469, "date/time string"=w468, "date/time string"=w467, "date/time string"=w466, "date/time string"=w465) -> (w439:T13)  [unwired: 1 in]
        n309 = Bundle("INCLUDED 4"="INCLUDED 4", "date/time string"=w415, "date/time string"=w414, "date/time string"=w413, "date/time string"=w412, "date/time string"=w411, "date/time string"=w410, "date/time string"=w409, "date/time string"=w408) -> (w407:T14)  [unwired: 1 in]
        n310 = Bundle("date/time string"=w452, "date/time string"=w451, "date/time string"=w450, "date/time string"=w449, "date/time string"=w448, "date/time string"=w447, "date/time string"=w446, "date/time string"=w445) -> (w425:T15)  [unwired: 1 in]
        n311 = Bundle("INCLUDED 6"="INCLUDED 6", "date/time string"=w396, "date/time string"=w395, "date/time string"=w394, "date/time string"=w393, "date/time string"=w392, "date/time string"=w391, "date/time string"=w390, "date/time string"=w389) -> (w397:T16)  [unwired: 1 in]
        n312 = Bundle("INCLUDED 5"="INCLUDED 5", "date/time string"=w406, "date/time string"=w405, "date/time string"=w404, "date/time string"=w403, "date/time string"=w402, "date/time string"=w401, "date/time string"=w400, "date/time string"=w399) -> (w398:T17)  [unwired: 1 in]
        n313 = Bundle("INCLUDED 2"="INCLUDED 2", "date/time string"=w464, "date/time string"=w463, "date/time string"=w462, "date/time string"=w461, "date/time string"=w460, "date/time string"=w459) -> (w435:T18)  [unwired: 1 in]
        n314 = Bundle("INCLUDED 3"="INCLUDED 3", "date/time string"=w458, "date/time string"=w457, "date/time string"=w456, "date/time string"=w455, "date/time string"=w454, "date/time string"=w453) -> (w429:T19)  [unwired: 1 in]
        n315 = call <vilib>:"DB Tools Update Data.vi"("condition"="where SNAME ='D3' ", "data"=w472, "error in (no error)"=w443, "columns"=string[] ["INCCLUDED", "AST", "AE", "BST", "BE", "CST", "CE"], "table"="SHIFT_TRAS", "connection reference"=w444) -> ("error out"=w436:errorcluster, "connection reference out"=w437:T4)  [unwired: 4 in]
        n316 = Bundle("Cycle_time(s)"="Cycle_time(s)") -> (w316:cluster{"Cycle_time(s)":dbl})  [unwired: 1 in]
        n317 = call <vilib>:"DB Tools Update Data.vi"("condition"="where SNAME ='B13' ", "data"=w439, "error in (no error)"=w436, "columns"=string[] ["INCCLUDED", "AST", "AE", "BST", "BE", "CST", "CE"], "table"="SHIFT_TRAS", "connection reference"=w437) -> ("error out"=w358:errorcluster, "connection reference out"=w359:T4)  [unwired: 4 in]
        n318 = call <vilib>:"DB Tools Update Data.vi"("condition"="where SNAME ='B23' ", "data"=w435, "error in (no error)"=w358, "columns"=string[] ["INCCLUDED", "AST", "AE", "BST", "BE", "CST", "CE"], "table"="SHIFT_TRAS", "connection reference"=w359) -> ("error out"=w356:errorcluster, "connection reference out"=w357:T4)  [unwired: 4 in]
        n319 = call <vilib>:"DB Tools Update Data.vi"("condition"="where SNAME ='B33' ", "data"=w429, "error in (no error)"=w356, "columns"=string[] ["INCCLUDED", "AST", "AE", "BST", "BE", "CST", "CE"], "table"="SHIFT_TRAS", "connection reference"=w357) -> ("error out"=w354:errorcluster, "connection reference out"=w355:T4)  [unwired: 4 in]
        n320 = call <vilib>:"DB Tools Update Data.vi"("condition"="where SNAME ='D4' ", "data"=w425, "error in (no error)"=w354, "columns"=string[] ["AST", "AE", "BST", "BE", "CST", "CE", "DST", "DE"], "table"="SHIFT_TRAS", "connection reference"=w355) -> ("error out"=w352:errorcluster, "connection reference out"=w353:T4)  [unwired: 4 in]
        n321 = call <vilib>:"DB Tools Update Data.vi"("condition"="where SNAME ='B14' ", "data"=w407, "error in (no error)"=w352, "columns"=string[] ["INCCLUDED", "AST", "AE", "BST", "BE", "CST", "CE", "DST", "DE"], "table"="SHIFT_TRAS", "connection reference"=w353) -> ("error out"=w350:errorcluster, "connection reference out"=w351:T4)  [unwired: 4 in]
        n322 = call <vilib>:"DB Tools Update Data.vi"("condition"="where SNAME ='B24' ", "data"=w398, "error in (no error)"=w350, "columns"=string[] ["INCCLUDED", "AST", "AE", "BST", "BE", "CST", "CE", "DST", "DE"], "table"="SHIFT_TRAS", "connection reference"=w351) -> ("error out"=w348:errorcluster, "connection reference out"=w349:T4)  [unwired: 4 in]
        n323 = call <vilib>:"DB Tools Update Data.vi"("condition"="where SNAME ='B34' ", "data"=w397, "error in (no error)"=w348, "columns"=string[] ["INCCLUDED", "AST", "AE", "BST", "BE", "CST", "CE", "DST", "DE"], "table"="SHIFT_TRAS", "connection reference"=w349) -> ("error out"=w346:errorcluster, "connection reference out"=w347:T4)  [unwired: 4 in]
        n324 = call <vilib>:"DB Tools Update Data.vi"("condition"="where SNAME ='D2' ", "data"=w370, "error in (no error)"=w346, "columns"=string[] ["INCCLUDED", "XST", "XE", "YST", "YE"], "table"="SHIFT_TRAS", "connection reference"=w347) -> ("error out"=w344:errorcluster, "connection reference out"=w345:T4)  [unwired: 4 in]
        n325 = call <vilib>:"DB Tools Update Data.vi"("condition"="where SNAME ='B12' ", "data"=w366, "error in (no error)"=w344, "columns"=string[] ["INCCLUDED", "XST", "XE", "YST", "YE"], "table"="SHIFT_TRAS", "connection reference"=w345) -> ("error out"=w342:errorcluster, "connection reference out"=w343:T4)  [unwired: 4 in]
        n326 = call <vilib>:"DB Tools Update Data.vi"("condition"="where SNAME ='B22' ", "data"=w363, "error in (no error)"=w342, "columns"=string[] ["INCCLUDED", "XST", "XE", "YST", "YE"], "table"="SHIFT_TRAS", "connection reference"=w343) -> ("error out"=w340:errorcluster, "connection reference out"=w341:T4)  [unwired: 4 in]
        n327 = call <vilib>:"DB Tools Update Data.vi"("condition"="where SNAME ='B32' ", "data"=w360, "error in (no error)"=w340, "columns"=string[] ["INCCLUDED", "XST", "XE", "YST", "YE"], "table"="SHIFT_TRAS", "connection reference"=w341) -> ("error out"=w321:errorcluster, "connection reference out"=w322:T4)  [unwired: 4 in]
        n328 = call <vilib>:"DB Tools Update Data.vi"("condition"="where SNAME ='Cycle' ", "data"=w316, "error in (no error)"=w321, "columns"=string[] ["time"], "table"="SHIFT_TRAS", "connection reference"=w322) -> ("error out"=w319:errorcluster, "connection reference out"=w320:T4)  [unwired: 4 in]
      }
      event "Cancel Button": Value Change {
        n329 = event-data() -> ()  [unwired: 1 in, 6 out]
      }
    }
  }
  n330 = call <vilib>:"DB Tools Close Connection.vi"("error in (no error)"=w282, "connection reference"=w283) -> ("error out"=w3:errorcluster)  [unwired: 5 in]
  n331 = call <vilib>:"Simple Error Handler.vi"("error in (no error)"=w3) -> ("error out"=w5:errorcluster)  [unwired: 4 in, 4 out]
  n332 = call <vilib>:"Clear Errors.vi"("error in (no error)"=w5) -> ("error out"=w4:errorcluster)  [unwired: 5 in, 1 out]
  n333 = flat-sequence {
    tunnel: w4 -> [w711]
    tunnel: [w711] -> w2
    tunnel: [w715] -> w6
    tunnel: w2 -> [w713]
    frame #0 {
      n334 = global write "Global 1.vi" "REMOVE VI"(TRUE ("remove_VI")) -> ()
    }
    frame #1 {
      n335 = property class="App"(error in=w713) -> (error out=w712:errorcluster, "App.Kind"=w714:T20)  [unwired: 1 in, 1 out]
      n336 = case shown="\"Run Time System\"" w714 {
        tunnel: [w716 w718] -> w715
        tunnel: w712 -> [w716 w717]
        frame "invalid app kind", Default {
        }
        frame "Run Time System" {
          n337 = disable-structure shown="Enabled" {
            disable-tunnel: [w720 _] -> w718
            disable-tunnel: w717 -> [w719 _]
            frame Enabled {
              n338 = invoke class="VI" method="FP.Close"(error in=w719) -> (error out=w720:errorcluster)  [unwired: 2 in, 2 out]
            }
            frame Disabled {
            }
          }
        }
      }
    }
  }
  "error out" <- w6
